vi "Process Tab Key.vi"(0 "MulticolumnListbox in":refnum<vi>, 5 "Columns":T1[](array[typedef]), 7 "increment":i32) -> ()   [LabVIEW 2020, in "KTable.xctl"]
uses:
  KTable.xctl
  ColumnSpec.ctl
  ColumnType.ctl
  Array Manipulation VIs/Array-Dimensions (2D string).vi
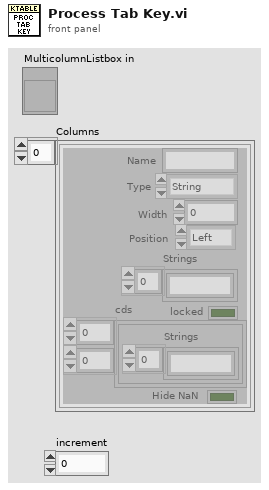
[diagram p1: front panel]
types:
  T1 = typedef "KTable.xctl/ColumnSpec.ctl" = cluster{"Name":string, "Type":T2, "Width":i32, "Strings":string[], "Position":enum16{"Left", "Center", "Right"}, "locked":bool, "cds":cluster{"Strings":string[]}[][], "Hide NaN":bool}
  T2 = typedef "KTable.xctl/ColumnType.ctl" = enum16{"String", "Enum", "Int", "Double", "Boolean", "Ring", "Formula", "Color"}
  T3 = typedef "LVRowAndColumnTypeDef.ctl" = cluster{"Row":i32, "Column":i32}
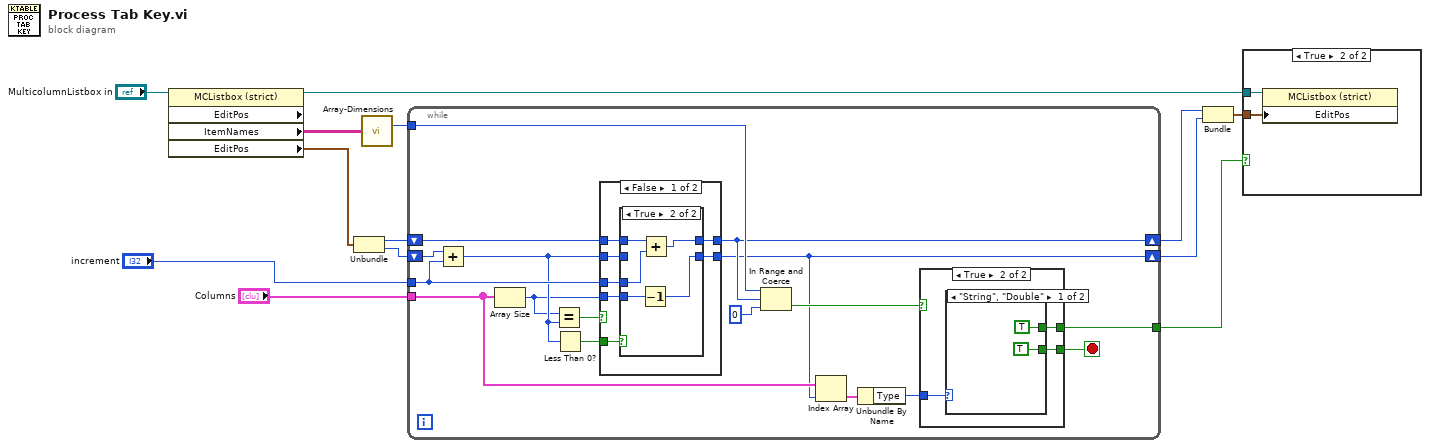
[diagram p0: block diagram]
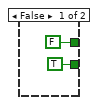
[diagram p3: hidden frame]
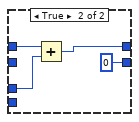
[diagram p6: hidden frame]
diagram:
  n1 = property class="MCListbox (strict)" props=["EditPos", "ItemNames", "EditPos"](reference="MulticolumnListbox in") -> (reference out=w12:refnum<vi>, "ItemNames"=w11:string[][], "EditPos"=w6:T3)  [unwired: 1 in, 2 out]
  n2 = Unbundle(w6) -> ("Row"=w10:i32, "Column"=w9:i32)
  n3 = call-poly "Array-Dimensions.vi"("2D Array"=w11) -> ("# rows"=w5:i32)  [unwired: 13 in, 1 out]
  n4 = while {
    shift-right: [w16] -> w4
    shift-left: w10 -> [w29]
    shift-right: [w14] -> w3
    shift-left: w9 -> [w30]
    tunnel: "increment" -> [w25]
    tunnel: "Columns" -> [w26]
    tunnel: w5 -> [w21]
    tunnel: [w17] -> w1
    stop <- w18 stop-if-true
    n5 = Add(x=w30, y=w25) -> (x+y=w24:i32)
    n6 = Array Size(array=w26) -> (size(s)=w22:i32)
    n7 = Equal?(x=w22, y=w24) -> (x = y?=w27:bool)
    n8 = Less Than 0?(x=w24) -> (x < 0?=w23:bool)
    n9 = case shown="False" w27 {
      tunnel: w24 -> [w40 _]
      tunnel: w29 -> [w42 w55]
      tunnel: w25 -> [w38 w54]
      tunnel: [w43 w53] -> w16
      tunnel: [w41 0] -> w14
      tunnel: w23 -> [w44 _]
      tunnel: w22 -> [w39 _]
      frame False {
        n10 = case shown="True" w44 {
          tunnel: [w46 w47] -> w43
          tunnel: w42 -> [w46 w49]
          tunnel: [w45 w50] -> w41
          tunnel: w40 -> [w45 _]
          tunnel: w39 -> [_ w51]
          tunnel: w38 -> [_ w48]
          frame False {
          }
          frame True {
            n11 = Decrement(x=w51) -> (x-1=w50:i32)
            n12 = Add(x=w49, y=w48) -> (x+y=w47:i32)
          }
        }
      }
      frame True {
        n13 = Add(x=w55, y=w54) -> (x+y=w53:i32)
      }
    }
    n14 = In Range and Coerce(upper limit=w21, x=w16, lower limit=0) -> (In Range?=w19:bool)  [unwired: 1 out]
    n15 = Index Array(array=w26, index=w14) -> (element=w28:T1)
    n16 = Unbundle By Name(w28) -> ("Type"=w15:T2)
    n17 = case shown="True" w19 {
      tunnel: [TRUE w34] -> w18
      tunnel: [FALSE w33] -> w17
      tunnel: w15 -> [_ w35]
      frame False {
      }
      frame True {
        n18 = case shown="\"String\", \"Double\"" w35 {
          tunnel: [TRUE _] -> w34
          tunnel: [TRUE _] -> w33
          frame "String", "Double" {
          }
          frame "Enum", Default {
          }
        }
      }
    }
  }
  n19 = Bundle("Row"=w4, "Column"=w3) -> (w2:cluster{"Row":i32, "Column":i32})  [unwired: 1 in]
  n20 = case shown="True" w1 {
    tunnel: w12 -> [_ w57]
    tunnel: w2 -> [_ w56]
    frame False {
    }
    frame True {
      n21 = property class="MCListbox (strict)"(reference=w57, "EditPos"=w56) -> ()  [unwired: 1 in, 2 out]
    }
  }
